vi "All Complex.vi"() -> (3 "GEMM Benchmark":cluster{i32[], dbl[]}[](graph))   [LabVIEW 2020]
doc: "Execute GEMM Process for different size on different Toolkits (Accelerator/Culab/CUDA/LabVIEW/G2CPU) and LabVIEW(CPU)."
uses:
  Source/_Controls/acc_execution_provider_enum.ctl
  <vilib>/Natan Biesmans/G2CPU GPU and CPU HPC Toolkit/ArrayFire Driver/TypeDefs/backend.ctl
  <vilib>/Natan Biesmans/G2CPU GPU and CPU HPC Toolkit/ArrayFire Driver/AF.lvlib
panel:
  out "Accelerator CUDA":bool
  out "Culab":bool
  out "Accelerator TRT":bool
  out "LabVIEW":bool
  out "G2CPU":bool
  out "G2CPU Time":dbl
  out "LabVIEW Time":dbl
  out "Accelerator CUDA Time":dbl
  out "Culab Time":dbl
  out "Accelerator TRT Time":dbl
  # "Complex Process"
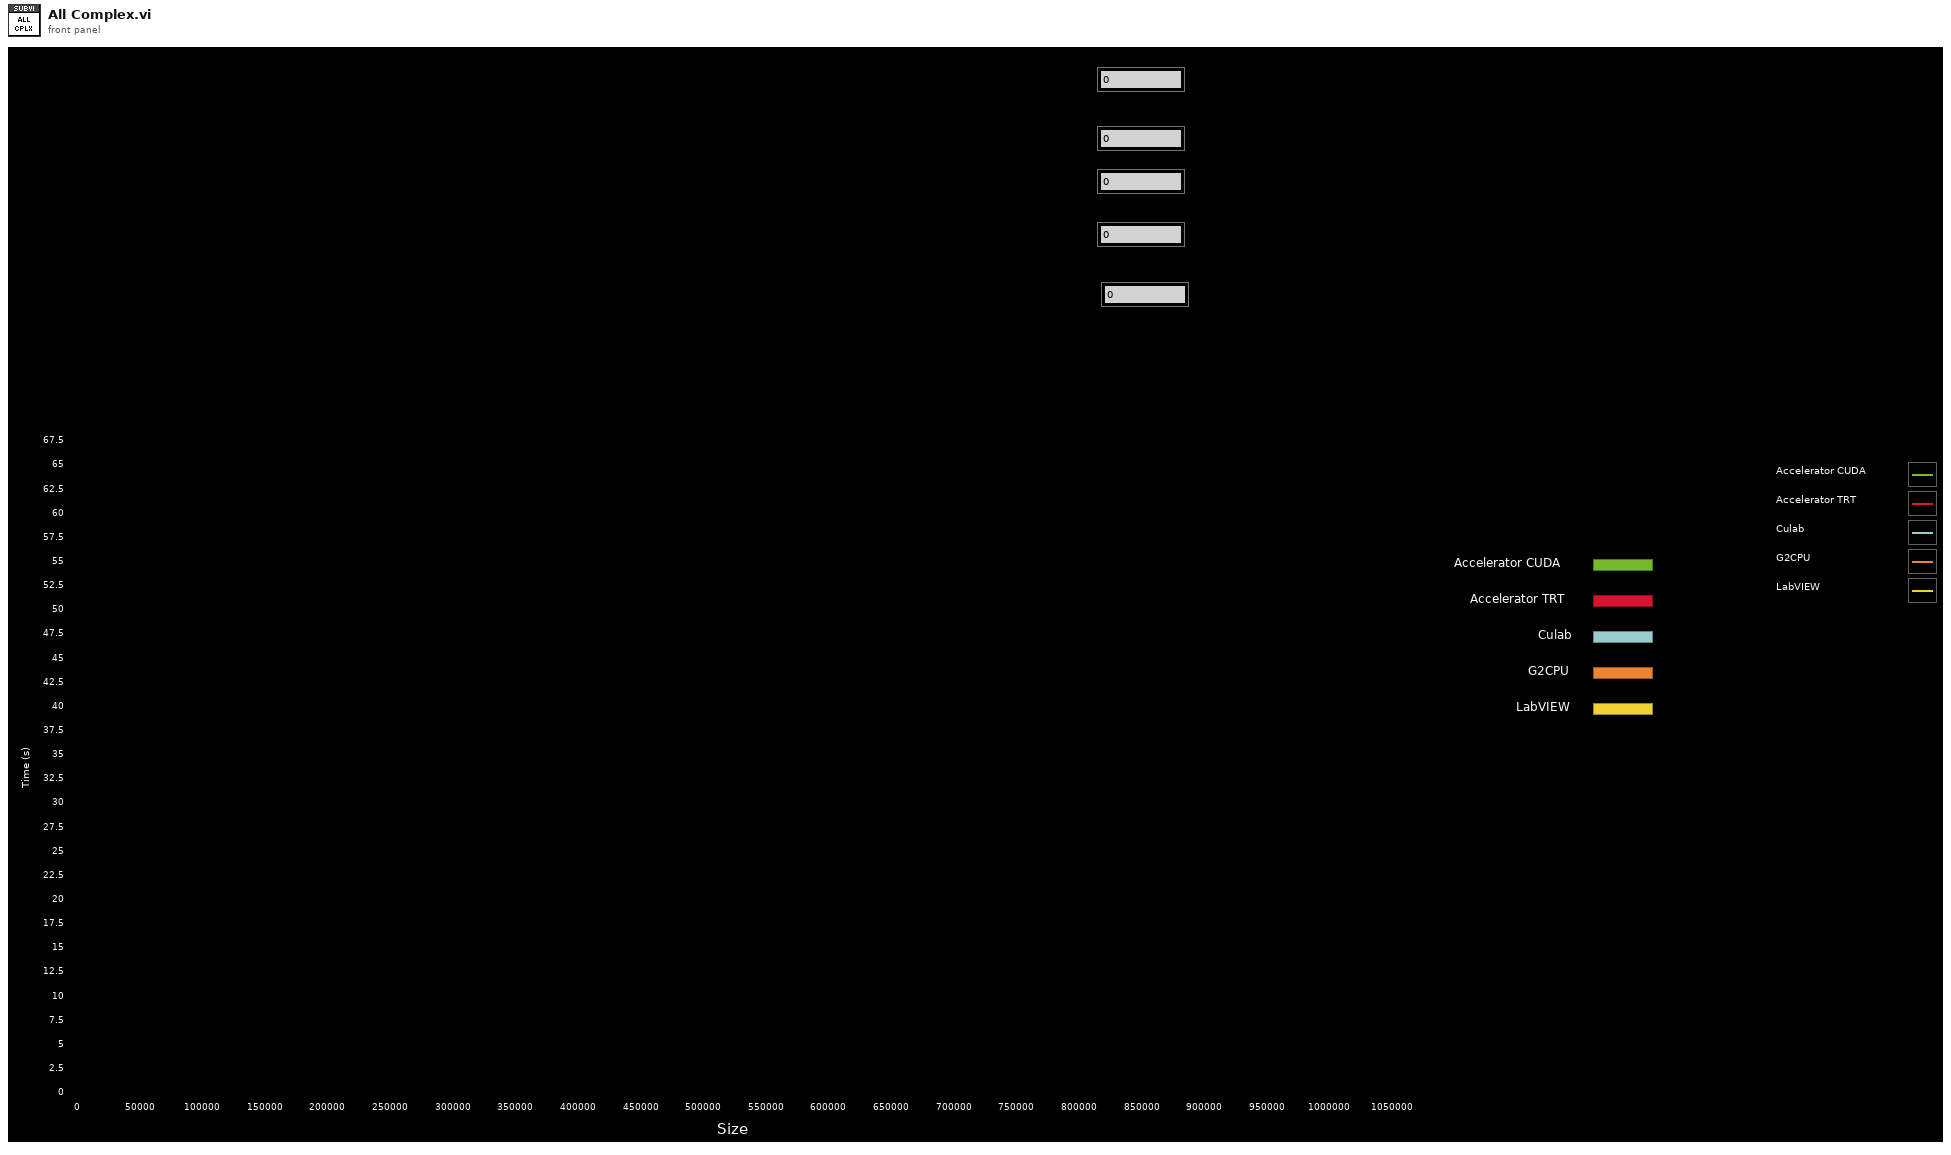
[diagram p1: front panel]
types:
  T1 = cluster{"intra_op_num_threads":i32, "inter_op_num_threads":i32, "execution_mode":enum16{"ORT_SEQUENTIAL", "ORT_PARALLEL"}, "deterministic_compute":bool, "graph_optimization_level":u16, "optimized_model_file_path":path, "profiling output dir":path}
  T2 = typedef "acc_execution_provider_enum.ctl" = enum16{"CPU", "CUDA", "TensorRT"}
  T3 = typedef "AF.lvlib/backend.ctl" = u32
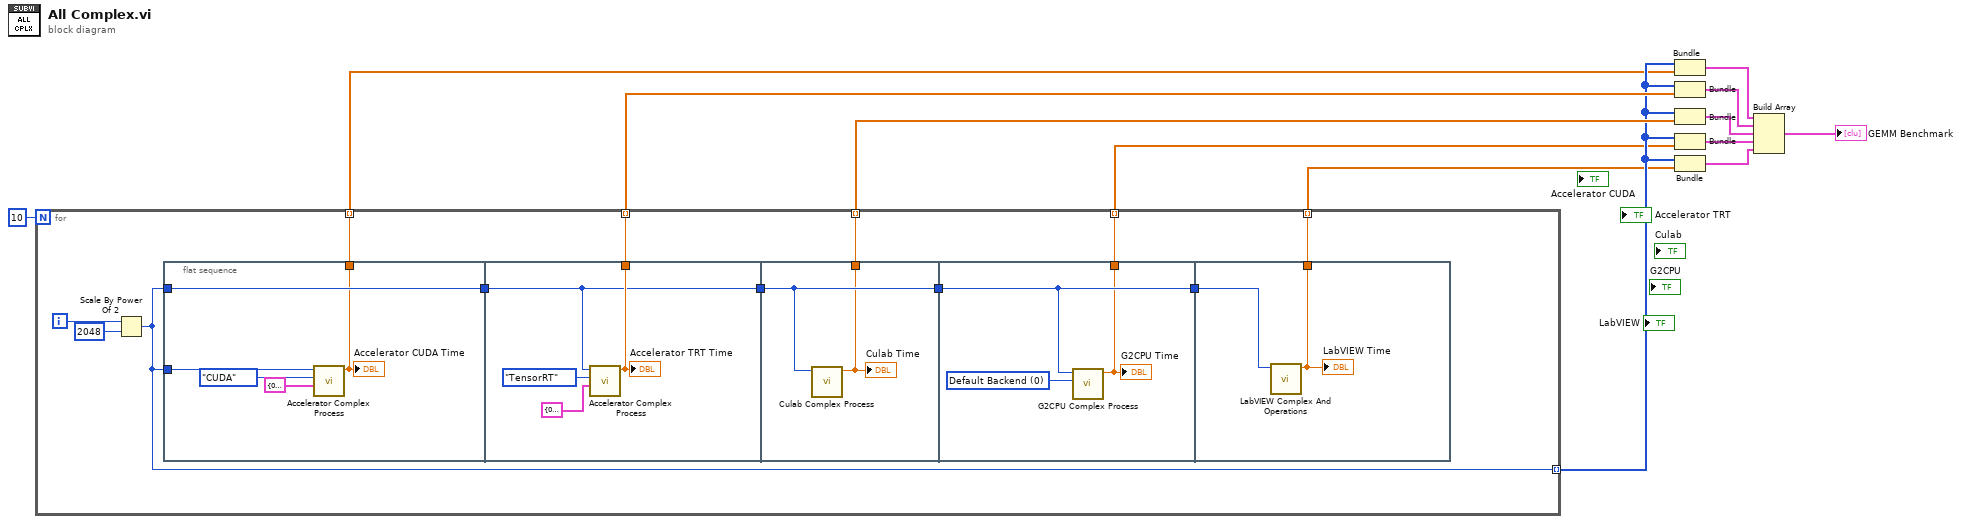
[diagram p0: block diagram]
diagram:
  n1 = for {
    N: 10 -> [_]
    tunnel: [w24] -> w12 mode=indexing
    tunnel: [w23] -> w11 mode=indexing
    tunnel: [w20] -> w6 mode=indexing
    tunnel: [w18] -> w3 mode=indexing
    tunnel: [w16] -> w5 mode=indexing
    tunnel: [w14] -> w2 mode=indexing
    i -> [w21]
    n2 = Scale By Power Of 2(n=w21, x=2048) -> (x*2^n=w20:i32)
    n3 = flat-sequence {
      tunnel: w20 -> [w30]
      tunnel: w20 -> [w28]
      tunnel: [w30] -> w17
      tunnel: [w27] -> w16
      tunnel: [w33] -> w25
      tunnel: [w34] -> w24
      tunnel: w17 -> [w33]
      tunnel: w25 -> [w36]
      tunnel: [w36] -> w15
      tunnel: [w35] -> w23
      tunnel: w15 -> [w39]
      tunnel: [w39] -> w19
      tunnel: [w38] -> w14
      tunnel: w19 -> [w40]
      tunnel: [w41] -> w18
      frame #0 {
        n4 = call "Accelerator Complex Process.vi"("Sessions Parameters"=T1 {"intra_op_num_threads"=0, "inter_op_num_threads"=0, "execution_mode"=enum."ORT_SEQUENTIAL", "deterministic_compute"=FALSE, "graph_optimization_level"=1, "optimized_model_file_path"=path "", "profiling output dir"=path ""}, "Execution Device"=acc_execution_provider_enum."CUDA", "X size"=w28) -> ("Accelerator Time"=w27:dbl)  [unwired: 8 in]
        "Accelerator CUDA Time" <- w27
      }
      frame #1 {
        n5 = call "Accelerator Complex Process.vi"("Sessions Parameters"=T1 {"intra_op_num_threads"=0, "inter_op_num_threads"=0, "execution_mode"=enum."ORT_SEQUENTIAL", "deterministic_compute"=FALSE, "graph_optimization_level"=1, "optimized_model_file_path"=path "", "profiling output dir"=path ""}, "Execution Device"=acc_execution_provider_enum."TensorRT", "X size"=w33) -> ("Accelerator Time"=w34:dbl)  [unwired: 8 in]
        "Accelerator TRT Time" <- w34
      }
      frame #2 {
        n6 = call "Culab Complex Process.vi"("X size"=w36) -> ("Culab Time"=w35:dbl)  [unwired: 10 in]
        "Culab Time" <- w35
      }
      frame #3 {
        w37 = T3 0 items=["Default Backend"=0, "CPU Backend"=1, "CUDA Backend"=2, "OPENCL Backend"=4, "Intel OneAPI Backend"=8] ("Backend")
        n7 = call "G2CPU Complex Process.vi"("Backend"=w37, "X size"=w39) -> ("G2CPU Time"=w38:dbl)  [unwired: 9 in]
        "G2CPU Time" <- w38
      }
      frame #4 {
        n8 = call "LabVIEW Complex And Operations.vi"("X size"=w40) -> ("LabVIEW Time"=w41:dbl)  [unwired: 10 in]
        "LabVIEW Time" <- w41
      }
    }
  }
  n9 = Bundle(w6, w5) -> (w7:cluster{i32[], dbl[]})  [unwired: 1 in]
  n10 = Bundle(w6, w12) -> (w8:cluster{i32[], dbl[]})  [unwired: 1 in]
  n11 = Bundle(w6, w11) -> (w10:cluster{i32[], dbl[]})  [unwired: 1 in]
  n12 = Bundle(w6, w2) -> (w4:cluster{i32[], dbl[]})  [unwired: 1 in]
  n13 = Bundle(w6, w3) -> (w1:cluster{i32[], dbl[]})  [unwired: 1 in]
  n14 = Build Array(w7, w8, w10, w4, w1) -> (→"GEMM Benchmark":cluster{i32[], dbl[]}[])
